vi "FP Position and Size.vi"(0 "VIRefNum  IN":refnum<vi>, 5 "Poistion":cluster{"left":i16, "top":i16}, 7 "Size":cluster{"right":i16, "bottom":i16}, 11 "error in (no error)":errorcluster, 12 "Mode":T1(ring)=enum."ALIGN -AS IS") -> (4 "VIRefNum OUT":refnum<vi>, 15 "error out":errorcluster)   [LabVIEW 2015]
panel:
  in  "Do Not Open FP":bool
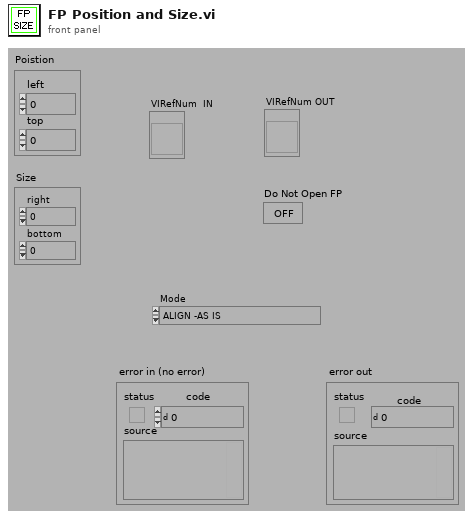
[diagram p1: front panel]
types:
  T1 = enum16{"ALIGN -CENTER", "ALIGN -TOP LEFT", "ALIGN -AS IS", "ALIGN -CUSTOM"}
  T2 = enum32{"Invalid", "Standard", "Closed", "Hidden", "Minimized", "Maximized"}
  T3 = typedef "LVRectTypeDef.ctl" = cluster{"Left":i16, "Top":i16, "Right":i16, "Bottom":i16}
  T4 = cluster{"left":i16, "top":i16, "right":i16, "bottom":i16}
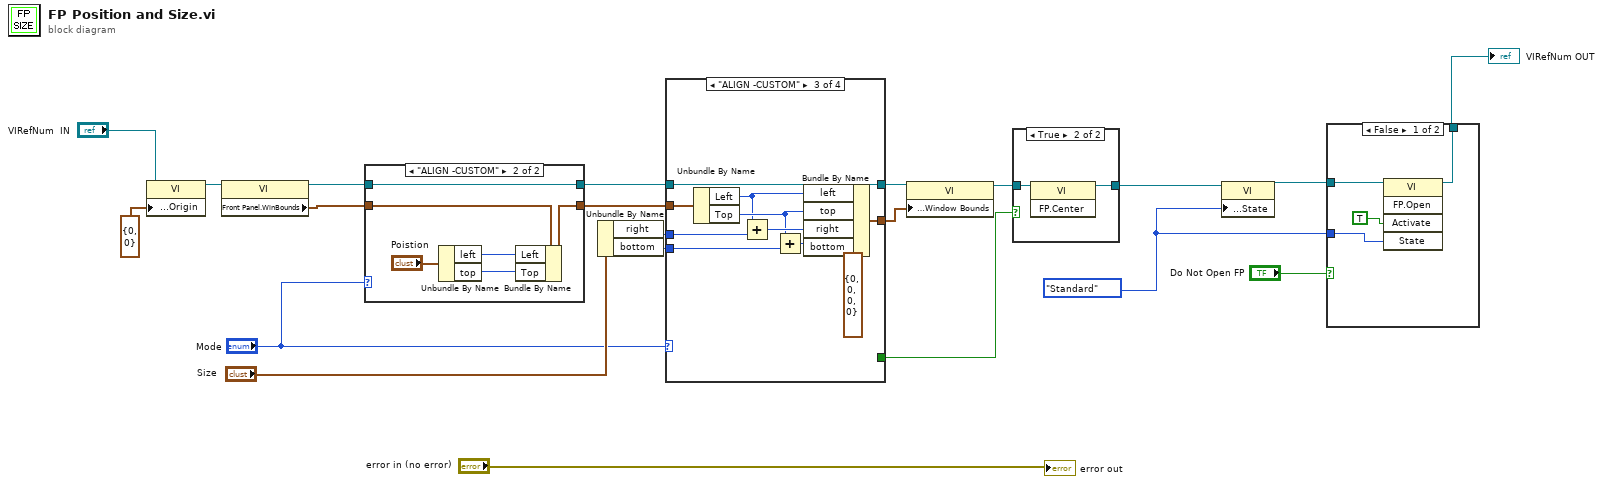
[diagram p0: block diagram]
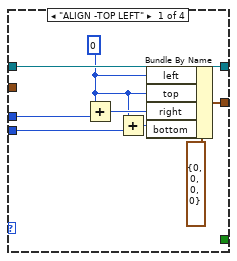
[diagram p5: hidden frame]
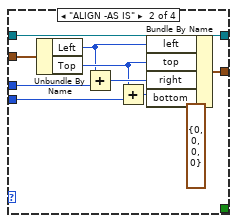
[diagram p6: hidden frame]
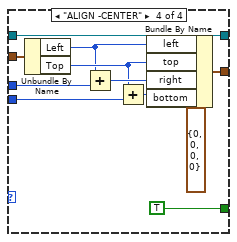
[diagram p7: hidden frame]
diagram:
  w4 = T2."Standard" ("Front Panel Window:State")
  n1 = property class="VI"(reference="VIRefNum  IN", "Front Panel Window:Origin"=cluster{"Horizontal":i16, "Vertical":i16} {"Horizontal"=0, "Vertical"=0}) -> (reference out=w11:refnum<vi>)  [unwired: 1 in, 1 out]
  n2 = property class="VI"(reference=w11) -> (reference out=w10:refnum<vi>, "Front Panel.WinBounds"=w9:T3)  [unwired: 1 in, 1 out]
  n3 = case shown="\"ALIGN -CUSTOM\"" "Mode" {
    tunnel: w10 -> [w23 w24]
    tunnel: [w23 w24] -> w7
    tunnel: w9 -> [w22 w26]
    tunnel: [w22 w25] -> w8
    frame Default {
    }
    frame "ALIGN -CUSTOM" {
      n4 = Unbundle By Name("Poistion") -> ("left"=w28:i16, "top"=w27:i16)
      n5 = Bundle By Name(cluster=w26, "Left"=w28, "Top"=w27) -> (w25:T3)
    }
  }
  n6 = Unbundle By Name("Size") -> ("right"=w16:i16, "bottom"=w18:i16)
  n7 = case shown="\"ALIGN -CUSTOM\"" "Mode" {
    tunnel: w18 -> [w37 w47 w57 w68]
    tunnel: w16 -> [w34 w43 w53 w64]
    tunnel: w8 -> [_ w40 w50 w61]
    tunnel: [w32 w39 w49 w60] -> w20
    tunnel: w7 -> [w31 w38 w48 w59]
    tunnel: [w31 w38 w48 w59] -> w21
    tunnel: [_ _ _ TRUE] -> w13
    frame "ALIGN -TOP LEFT" {
      w30 = i16 0 ("left")
      n8 = Add(x=w30, y=w34) -> (x+y=w35:i16)
      n9 = Add(x=w30, y=w37) -> (x+y=w36:i16)
      n10 = Bundle By Name(cluster=T4 {"left"=0, "top"=0, "right"=0, "bottom"=0} ("Front Panel Window:Panel Bounds"), "left"=w30, "top"=w30, "right"=w35, "bottom"=w36) -> (w32:T4)
    }
    frame "ALIGN -AS IS" {
      n11 = Unbundle By Name(w40) -> ("Left"=w42:i16, "Top"=w44:i16)
      n12 = Add(x=w42, y=w43) -> (x+y=w45:i16)
      n13 = Add(x=w44, y=w47) -> (x+y=w46:i16)
      n14 = Bundle By Name(cluster=T4 {"left"=0, "top"=0, "right"=0, "bottom"=0} ("Front Panel Window:Panel Bounds"), "left"=w42, "top"=w44, "right"=w45, "bottom"=w46) -> (w39:T4)
    }
    frame "ALIGN -CUSTOM" {
      n15 = Unbundle By Name(w50) -> ("Left"=w52:i16, "Top"=w54:i16)
      n16 = Add(x=w52, y=w53) -> (x+y=w55:i16)
      n17 = Add(x=w54, y=w57) -> (x+y=w56:i16)
      n18 = Bundle By Name(cluster=T4 {"left"=0, "top"=0, "right"=0, "bottom"=0} ("Front Panel Window:Panel Bounds"), "left"=w52, "top"=w54, "right"=w55, "bottom"=w56) -> (w49:T4)
    }
    frame "ALIGN -CENTER" {
      n19 = Unbundle By Name(w61) -> ("Left"=w63:i16, "Top"=w65:i16)
      n20 = Add(x=w63, y=w64) -> (x+y=w66:i16)
      n21 = Add(x=w65, y=w68) -> (x+y=w67:i16)
      n22 = Bundle By Name(cluster=T4 {"left"=0, "top"=0, "right"=0, "bottom"=0} ("Front Panel Window:Panel Bounds"), "left"=w63, "top"=w65, "right"=w66, "bottom"=w67) -> (w60:T4)
    }
  }
  n23 = property class="VI"(reference=w21, "Front Panel Window:Window Bounds"=w20) -> (reference out=w15:refnum<vi>)  [unwired: 1 in, 1 out]
  n24 = case shown="True" w13 {
    tunnel: w15 -> [w69 w71]
    tunnel: [w69 w70] -> w14
    frame False {
    }
    frame True {
      n25 = invoke class="VI" method="FP.Center"(reference=w71) -> (reference out=w70:refnum<vi>)  [unwired: 2 in, 2 out]
    }
  }
  n26 = property class="VI"(reference=w14, "Front Panel Window:State"=w4) -> (reference out=w6:refnum<vi>)  [unwired: 1 in, 1 out]
  n27 = case shown="False" "Do Not Open FP" {
    tunnel: w6 -> [w75 w76]
    tunnel: [w74 w76] -> w5
    tunnel: w4 -> [w73 _]
    frame False {
      n28 = invoke class="VI" method="FP.Open"(reference=w75, "Activate"=TRUE ("Activate?"), "State"=w73) -> (reference out=w74:refnum<vi>)  [unwired: 2 in, 4 out]
    }
    frame True {
    }
  }
  "VIRefNum OUT" <- w5
  "error out" <- "error in (no error)"
